vi "SQLite Select All SensorConfigValue_Old.vi"(6 "ALL/Single":T1(ring), 7 "Main":string="0", 8 "error in (no error)":errorcluster, 11 "SensorName":string) -> (0 "error out":errorcluster, 1 "SensorNameList":string[](array[string]), 2 "RowsNumber":string[](array[string]), 3 "Results":string[][](table), 5 "ColumnNames":string[](array[string]))   [LabVIEW 2015, in "SQLite.lvclass"]
doc: "读取Sensor的配置数据。\n2020-03-06 09:56:51\n蒋松\njiangsong@outlook.com"
uses:
  SQLite.lvclass
  SQLiteFileName.ctl
  TabelFullName.ctl
  <vilib>/Utility/error.llb/Trim Whitespace.vi
  <userlib>/sushu/sushu.lvlib
  <userlib>/LabSQL/LabSQL.lvlib
panel:
  out "resulting string":string
  out "OK？":bool
  out "Select SQL CMD":string
  out "String":string
  in  "error in (no error) 2":errorcluster
  # "8"
  # "8"
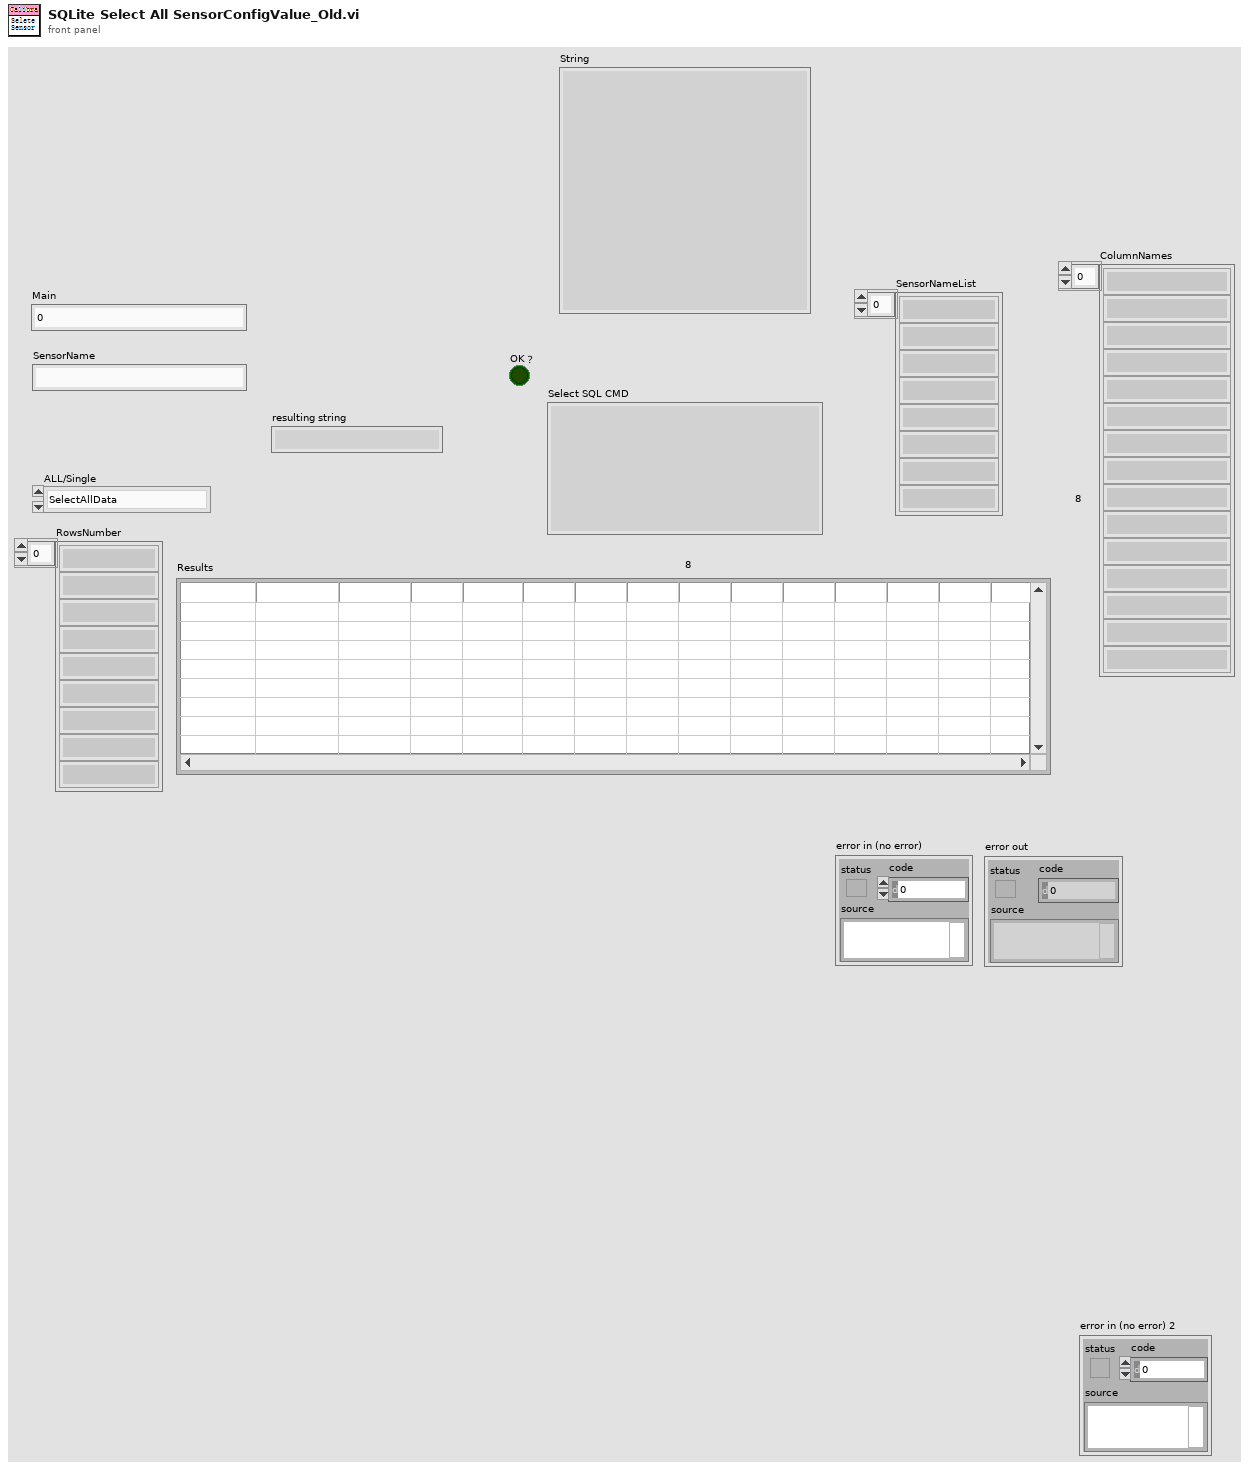
[diagram p1: front panel]
types:
  T1 = enum16{"SelectAllData", "SelectDataBySensorName"}
  T2 = typedef "SQLite.lvclass/TabelFullName.ctl" = string
  T3 = typedef "SQLite.lvclass/SQLiteFileName.ctl" = string
  T4 = enum16{"Other", "SQL2008", "SQLite", "Access", "MySQL"}
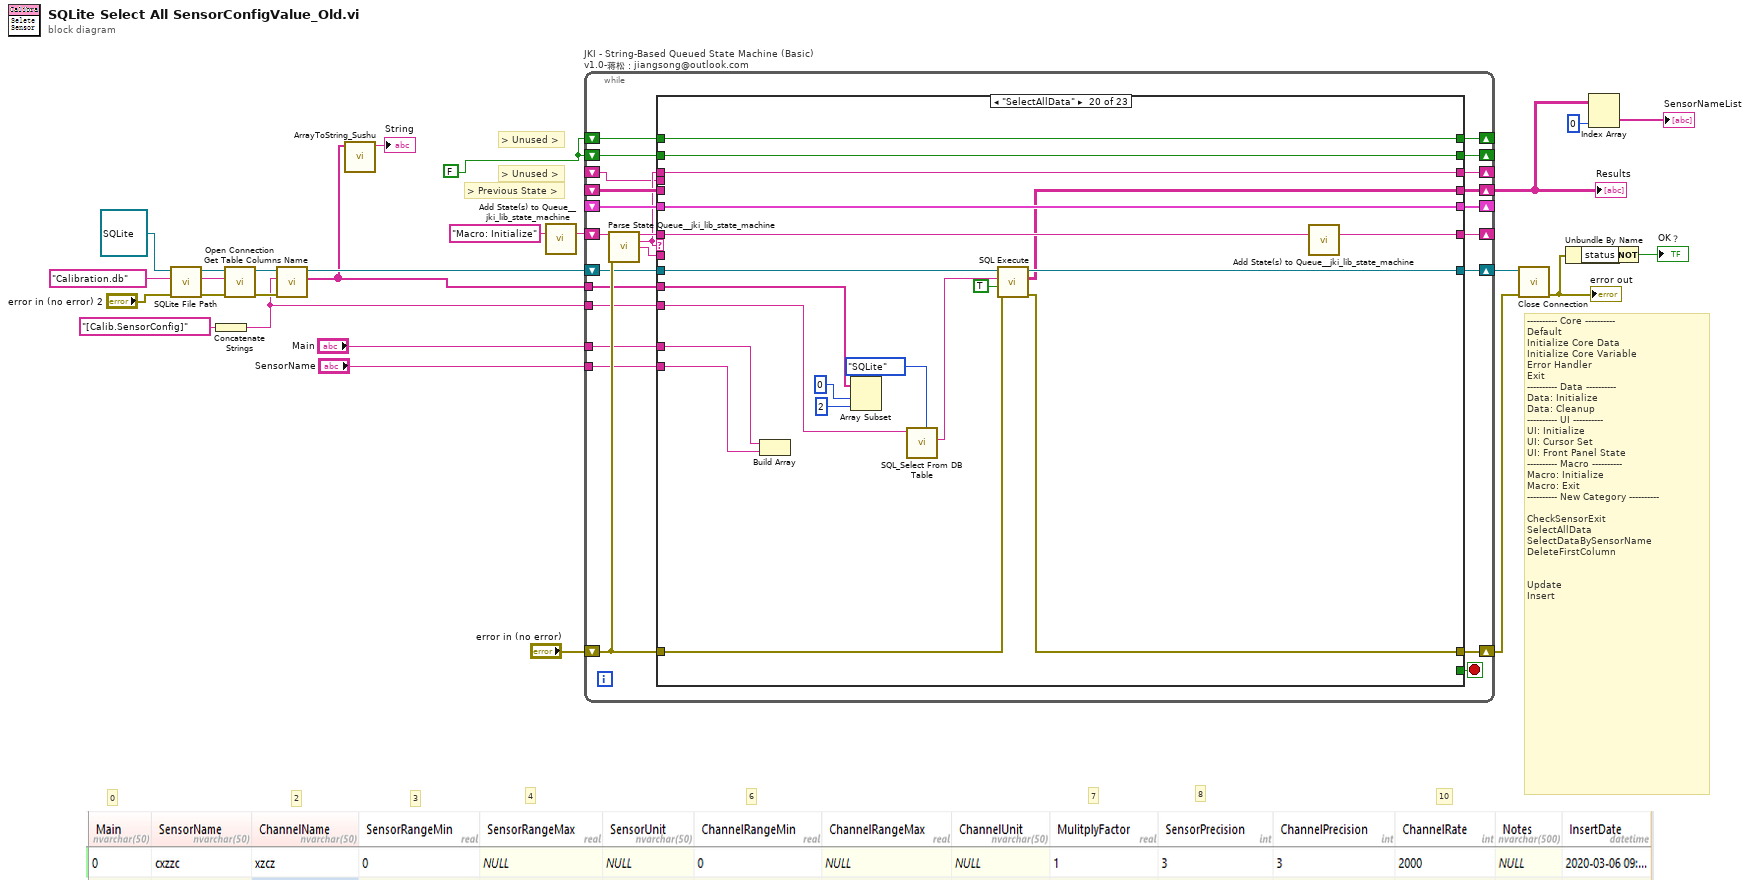
[diagram p0: block diagram]
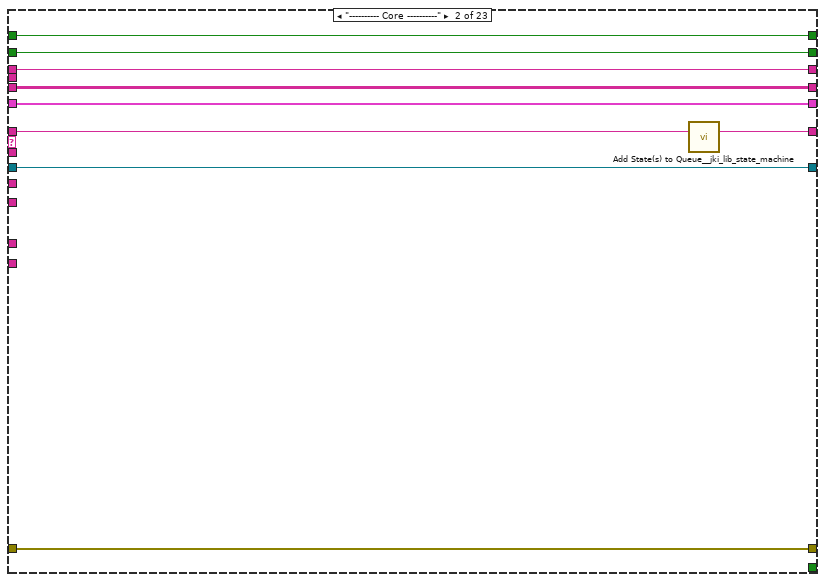
[diagram p3: hidden frame]
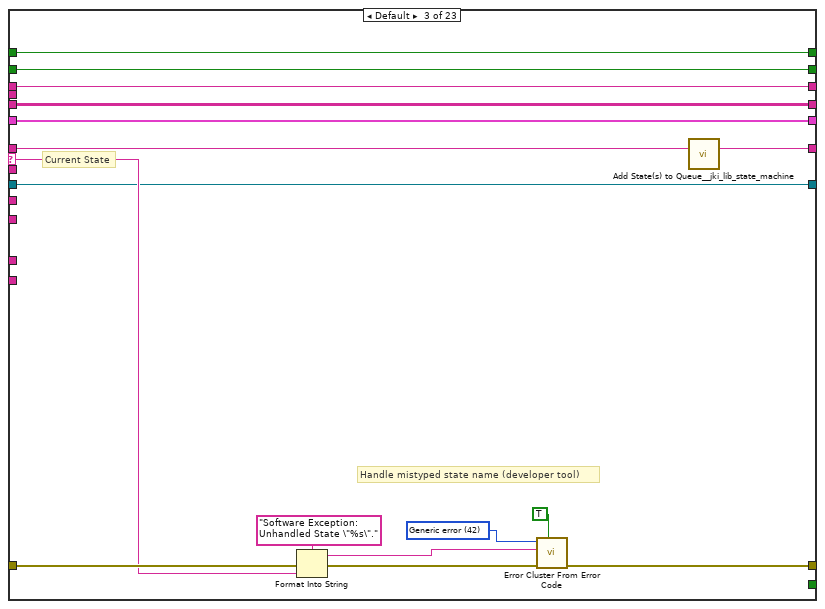
[diagram p4: hidden frame]
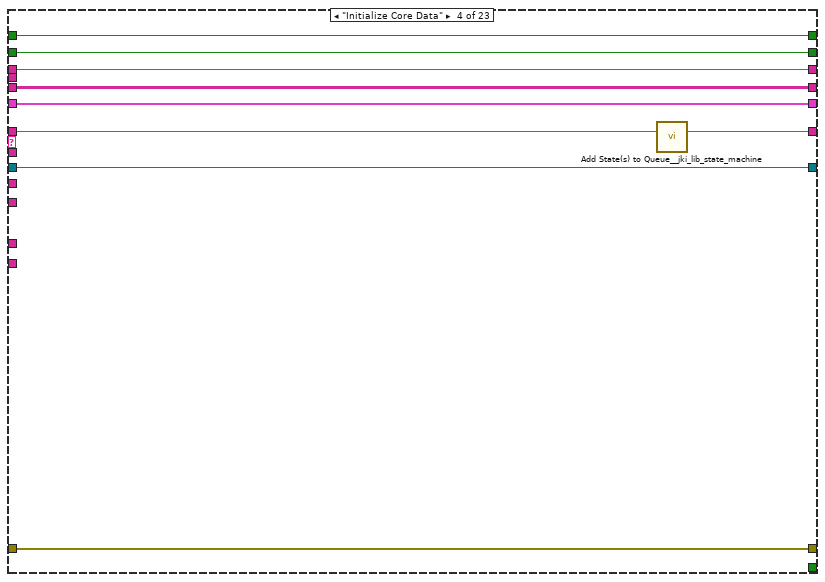
[diagram p5: hidden frame]
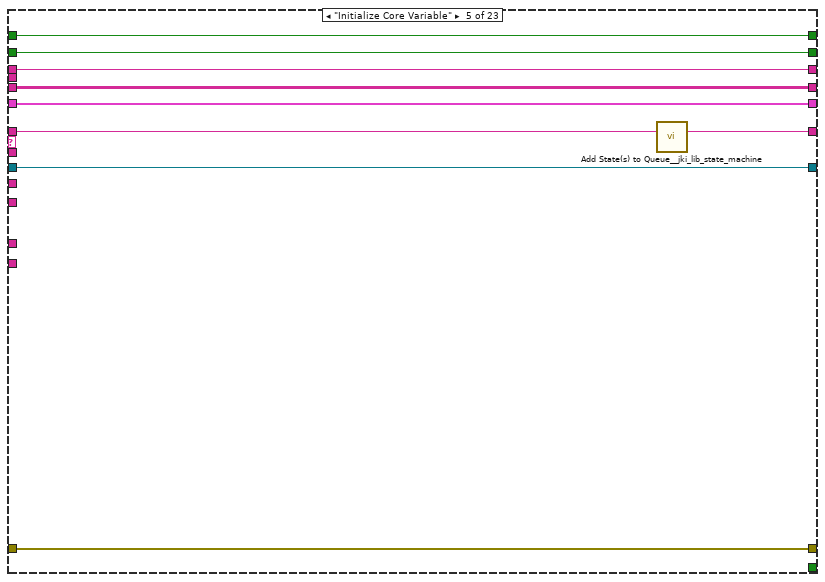
[diagram p6: hidden frame]
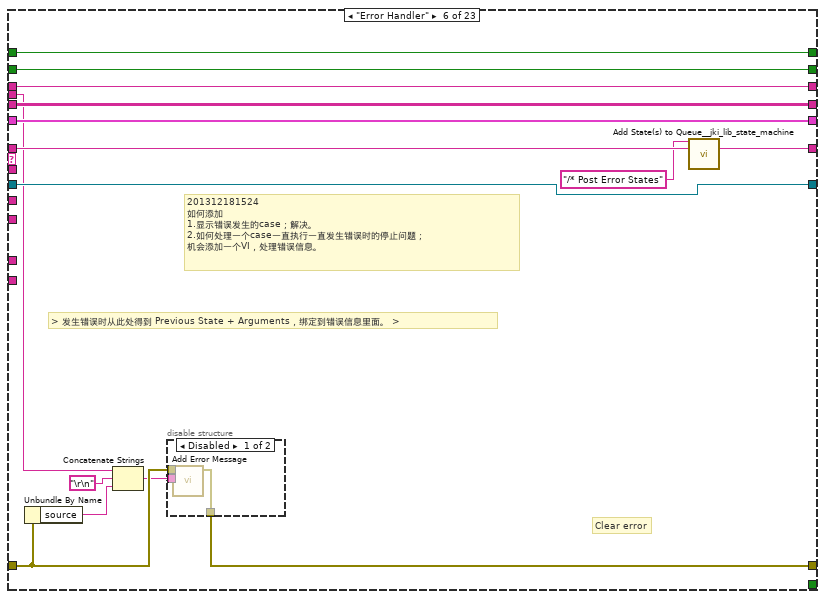
[diagram p7: hidden frame]
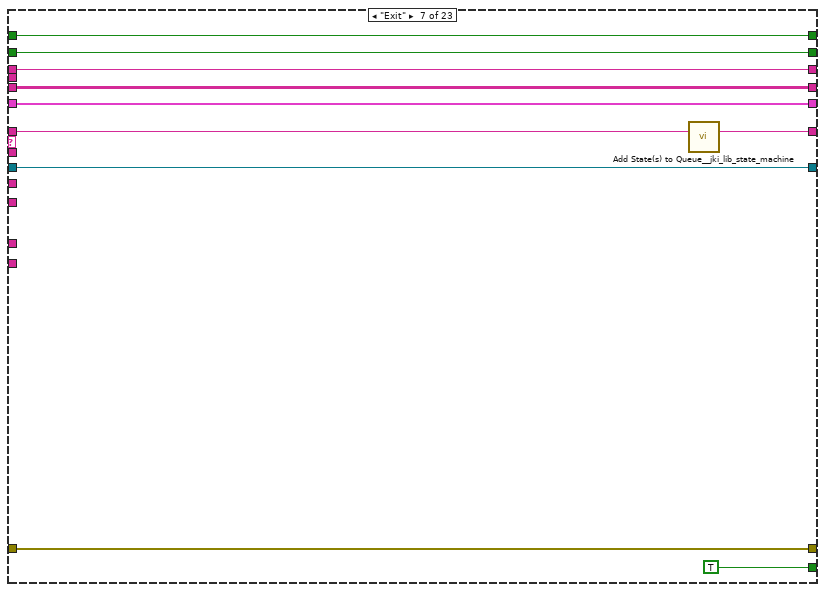
[diagram p9: hidden frame]
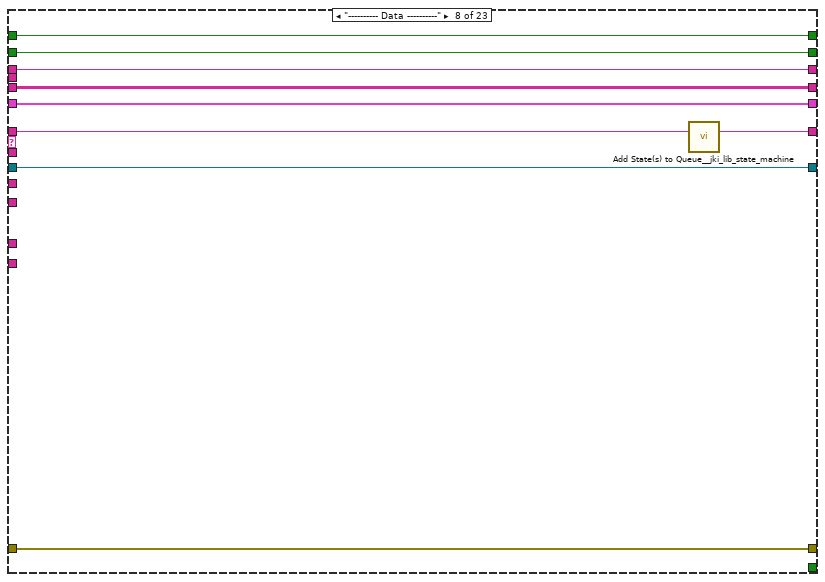
[diagram p10: hidden frame]
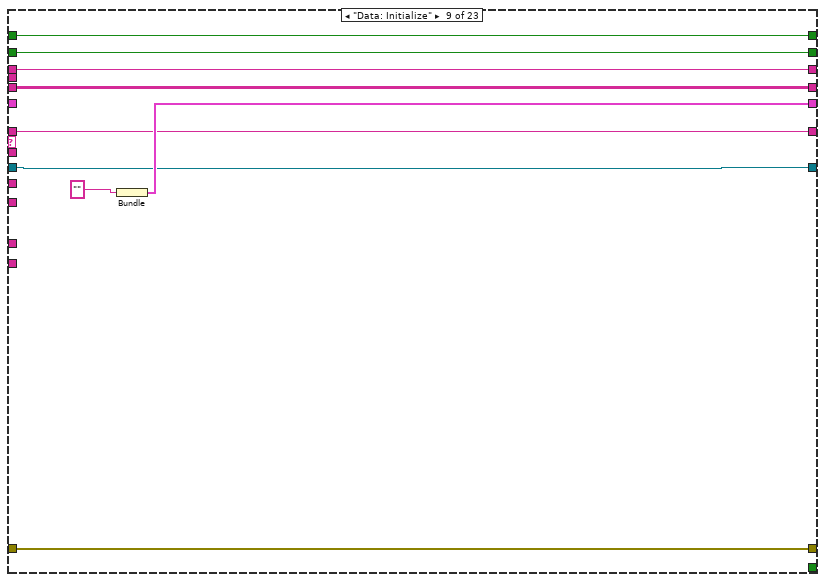
[diagram p11: hidden frame]
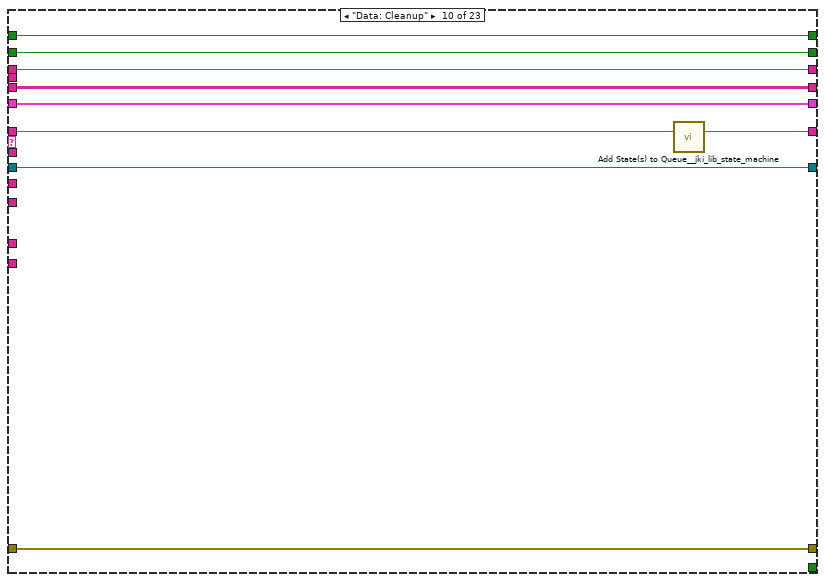
[diagram p12: hidden frame]
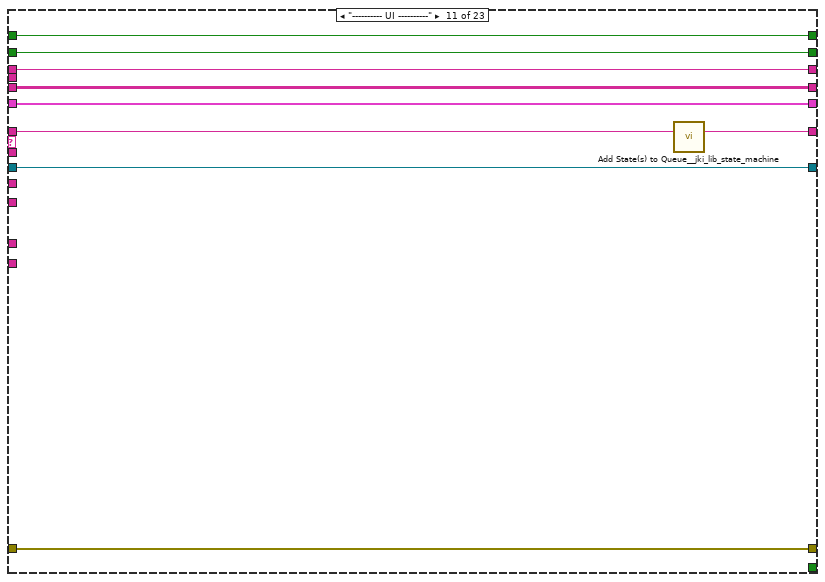
[diagram p13: hidden frame]
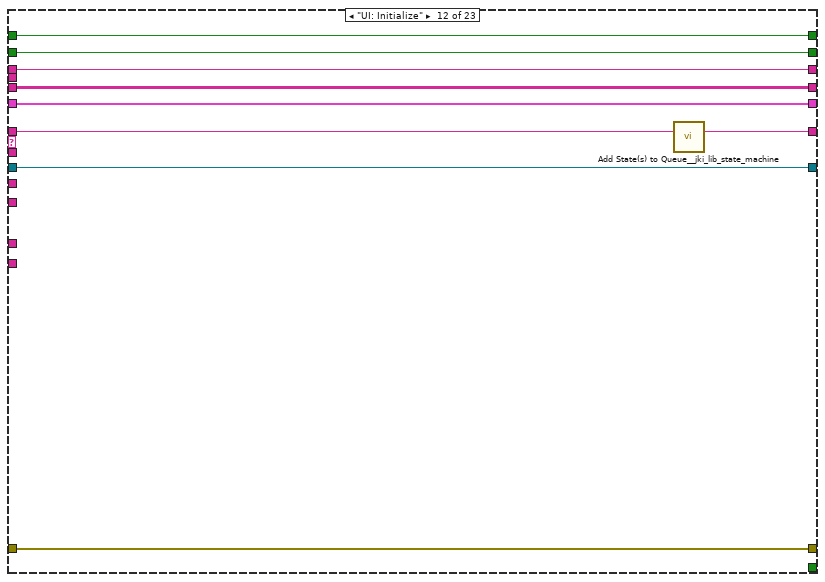
[diagram p14: hidden frame]
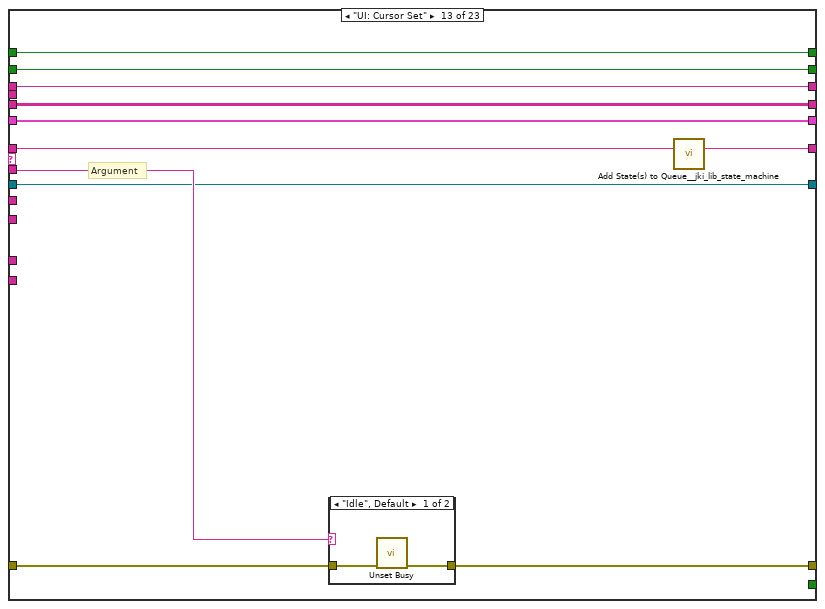
[diagram p15: hidden frame]
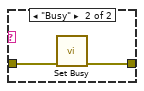
[diagram p16: hidden frame]
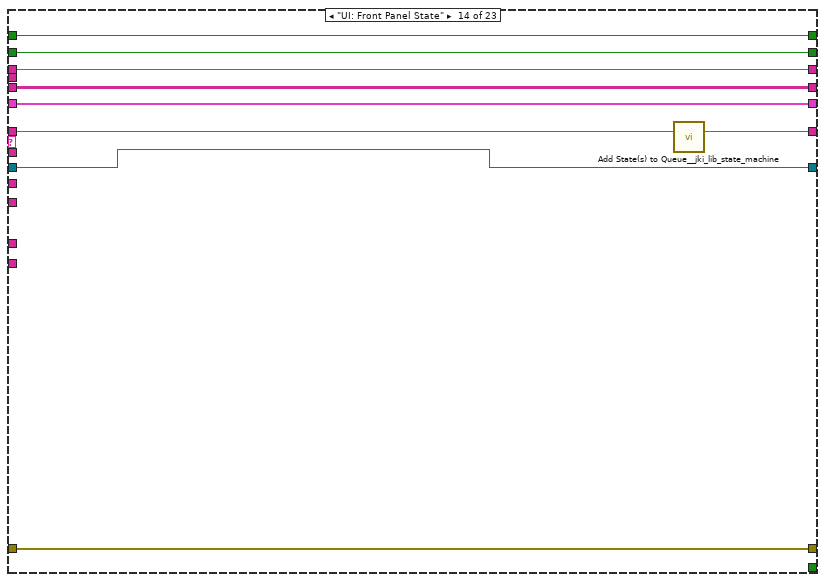
[diagram p17: hidden frame]
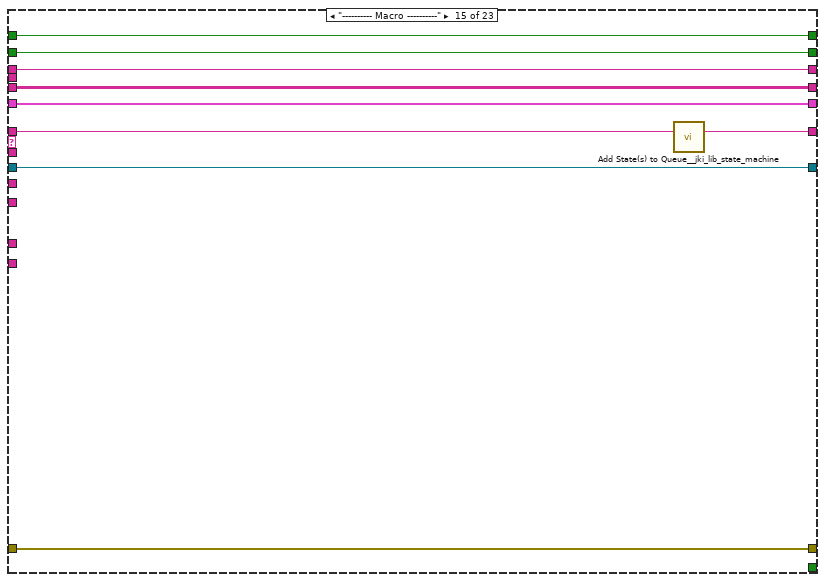
[diagram p18: hidden frame]
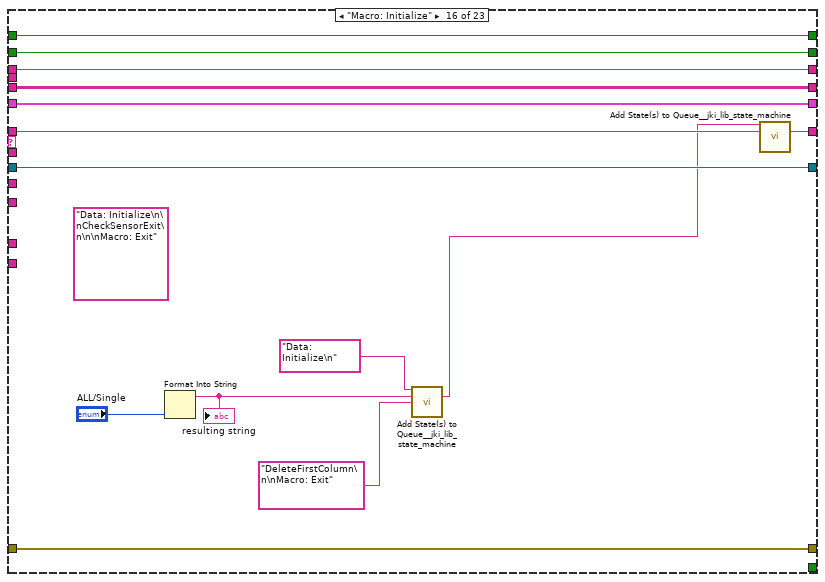
[diagram p19: hidden frame]
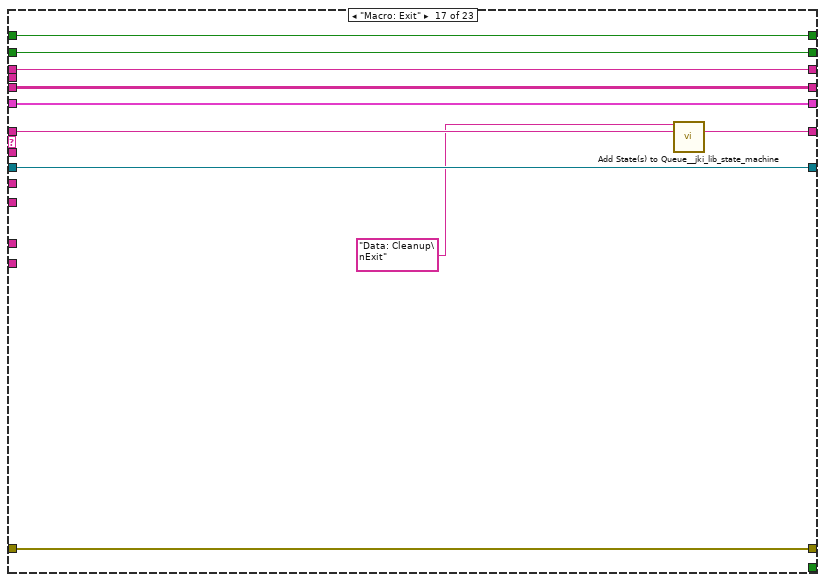
[diagram p20: hidden frame]
diagram:
  w4 = FALSE
  # "10"
  # "8"
  # "7"
  # "6"
  # "3"
  # "0"
  # "> Previous State >"
  # "> Unused >"
  # "> Unused >"
  # "---------- Core ----------\nDefault\nInitialize Core Data\nInitialize Core Variable\nError Handler\nExit\n---------- Data ----------\nData: Initialize\nData: Cleanup\n---------- UI ----------\nUI: Initialize\nUI: Cursor Set\nUI: Front Panel State\n---------- Macro ----------\nMacro: Initialize\nMacro: Exit\n---------- New Category ----------\n\nCheckSensorExit\nSelectAllData\nSelectDataBySensorName\nDeleteFirstColumn\n\n\nUpdate\nInsert"
  # "2"
  # "4"
  n1 = call "SQLite File Path.vi"("error in (no error)"="error in (no error) 2", "SQLiteFileName"=T3 "Calibration.db", "SQLite in"=refnum<class "SQLite.lvclass"> refnum ("SQLite.lvclass")) -> ("error out"=w22:errorcluster, "string"=w18:string, "SQLite out"=w20:refnum<class "SQLite.lvclass">)  [unwired: 6 in]
  n2 = Concatenate Strings(T2 "[Calib.SensorConfig]" ("TabelFullName")) -> (w13:string)
  n3 = call-dynamic "Open Connection.vi"("error in (no error)"=w22, "ConnectionString"=w18, "HostDB in"=w20) -> ("error out"=w17:errorcluster, "HostDB out"=w16:refnum<class "SQLite.lvclass">)  [unwired: 7 in]
  n4 = call-dynamic "Get Table Columns Name.vi"("error in (no error)"=w17, "TableName"=w13, "HostDB in"=w16) -> ("ColunmsList"=w9:string[], "HostDB out"=w14:refnum<class "SQLite.lvclass">)  [unwired: 4 in, 3 out]
  n5 = call <userlib>:"ArrayToString_Sushu.vi"("Array"=w9) -> ("String"=→"String":string)  [unwired: 10 in]
  n6 = call <vilib>:"Add State(s) to Queue__jki_lib_state_machine.vi"("State(s) in (\"\")"="Macro: Initialize") -> ("States Out"=w27:string)  [unwired: 14 in]
  n7 = while "JKI - String-Based Queued State Machine (Basic) v1.0-蒋松：jiangsong@outlook.com" {
    shift-right: [w49] -> w10
    shift-left: "error in (no error)" -> [w47]
    shift-right: [w30] -> _
    shift-left: w27 -> [w38]
    shift-right: [w43] -> _
    shift-left: w4 -> [w45]
    shift-right: [w44] -> _
    shift-left: w4 -> [w46]
    shift-right: [w39] -> _
    shift-left: _ -> [w42]
    shift-right: [w40] -> w3
    shift-left: _ -> [w31]
    shift-right: [w41] -> _
    shift-left: _ -> [w28]
    tunnel: w9 -> [w37]
    tunnel: w13 -> [w36]
    tunnel: "Main" -> [w35]
    tunnel: "SensorName" -> [w34]
    shift-right: [w32] -> w12
    shift-left: w14 -> [w33]
    stop <- w48 stop-if-true
    n8 = call <vilib>:"Parse State Queue__jki_lib_state_machine.vi"("State Queue"=w38, "Error In (no error)"=w47) -> ("Remaining States"=w51:string, "Current State"=w29:string, "Arguments"=w50:string)  [unwired: 11 in]
    n9 = case shown="\"SelectAllData\"" w29 {
      selector: w29 -> [_ _ w70 _ _ _ _ _ _ _ _ _ _ _ _ _ _ _ _ _ _ _ _]
      tunnel: w51 -> [w52 w68 w84 w93 w102 w117 w130 w139 w140 w157 w166 w175 w186 w199 w208 w214 w232 w241 w247 w269 w306 w332 w360]
      tunnel: w50 -> [_ _ _ _ _ _ _ _ _ _ _ _ w180 _ _ _ _ _ _ _ _ _ _]
      tunnel: [w59 w66 w71 w88 w100 w104 w123 w133 w145 w149 w160 w169 w178 w191 w202 w218 w227 w236 w245 w267 w307 w311 w335] -> w49
      tunnel: w47 -> [w59 w66 w72 w88 w100 w107 w123 w133 w145 w149 w160 w169 w179 w191 w202 w218 w227 w236 w246 w268 w307 w312 w336]
      tunnel: [w52 w67 w83 w92 w101 w116 w129 w138 w140 w156 w165 w174 w185 w198 w207 w215 w231 w240 w248 w270 w306 w332 w360] -> w30
      tunnel: [_ _ _ _ _ _ TRUE _ _ _ _ _ _ _ _ _ _ _ _ _ _ _ _] -> w48
      tunnel: w46 -> [w58 w65 w82 w91 w94 w115 w128 w137 w148 w155 w164 w173 w184 w197 w206 w222 w230 w239 w263 w283 w305 w331 w359]
      tunnel: w45 -> [w57 w64 w81 w90 w95 w114 w127 w136 w147 w154 w163 w172 w183 w196 w205 w221 w229 w238 w262 w282 w304 w330 w358]
      tunnel: [w58 w65 w82 w91 w94 w115 w128 w137 w148 w155 w164 w173 w184 w197 w206 w222 w230 w239 w263 w283 w305 w331 w359] -> w44
      tunnel: [w57 w64 w81 w90 w95 w114 w127 w136 w147 w154 w163 w172 w183 w196 w205 w221 w229 w238 w262 w282 w304 w330 w358] -> w43
      tunnel: w29 -> [w56 w63 w80 w89 w96 w113 w126 w135 w146 w153 w162 w171 w182 w195 w204 w220 w228 w237 w261 w281 w303 w329 w357]
      tunnel: w31 -> [w54 w61 w79 w87 w97 w110 w122 w132 w143 w151 w159 w168 w177 w193 w201 w217 w225 w234 _ _ w300 w328 w356]
      tunnel: w42 -> [w55 w62 w78 w85 w99 w105 w125 w134 _ w152 w161 w170 w181 w194 w203 w219 w226 w235 w260 w280 w302 w327 w355]
      tunnel: [w56 w63 w80 w89 w96 w113 w126 w135 w146 w153 w162 w171 w182 w195 w204 w220 w228 w237 w261 w281 w303 w329 w357] -> w41
      tunnel: [w54 w61 w79 w87 w97 w110 w122 w132 w143 w151 w159 w168 w177 w193 w201 w217 w225 w234 w244 w266 w287 w328 w356] -> w40
      tunnel: [w55 w62 w78 w85 w99 w105 w125 w134 w144 w152 w161 w170 w181 w194 w203 w219 w226 w235 w260 w280 w302 w327 w355] -> w39
      tunnel: w37 -> [_ _ _ _ _ _ _ _ _ _ _ _ _ _ _ _ _ _ w252 w274 w295 w319 w342]
      tunnel: w36 -> [_ _ _ _ _ _ _ _ _ _ _ _ _ _ _ _ _ _ w251 w273 _ w321 w348]
      tunnel: w35 -> [_ _ _ _ _ _ _ _ _ _ _ _ _ _ _ _ _ _ w250 w272 _ w326 w354]
      tunnel: w34 -> [_ _ _ _ _ _ _ _ _ _ _ _ _ _ _ _ _ _ w249 w271 _ w325 w353]
      tunnel: w33 -> [w53 w60 w69 w86 w98 w108 w121 w131 w142 w150 w158 w167 w176 w192 w200 w216 w224 w233 w254 w276 w301 w324 w352]
      tunnel: [w53 w60 w69 w86 w98 w108 w121 w131 w142 w150 w158 w167 w176 w192 w200 w216 w224 w233 w253 w275 w301 w323 w351] -> w32
      tunnel: w28 -> [_ _ _ _ _ w103 _ _ _ _ _ _ _ _ _ _ _ _ _ _ _ _ _]
      frame "Idle" {
      }
      frame "---------- Core ----------" {
        n10 = call <vilib>:"Add State(s) to Queue__jki_lib_state_machine.vi"("State(s) in (\"\")"=w68) -> ("States Out"=w67:string)  [unwired: 14 in]
      }
      frame Default {
        w74 = 42 items=["No error", "Argument error", "Memory is full", "Out of zone", "End of file", "File already open", "Generic file I/O error", "File not found", "File permission error", "Disk is full", "Duplicate path", "Too many files open", "System feature not enabled", "Resource file not found", "Cannot add resource", "Resource not found", "Image not found", "Image memory error", "Pen does not exist", "Config type invalid", "Config token not found", "Config parse error", "Config memory error", "Bad external code format", "Bad external code offset", "External code not present", "Null window", "Destroy window error", "Null menu", "Print aborted", "Bad print record", "Print driver error", "Windows error during printing", "Memory error during printing", "Print dialog error", "Generic print error", "Invalid device refnum", "Device not found", "Device parameter error", "Device unit error", "Cannot open device", "Device call aborted", "Generic error", "Cancelled by user", "Object ID too low", "Object ID too high", "Object not in heap", "Unknown heap", "Unknown object (invalid DefProc)", "Unknown object (DefProc not in table)", "Message out of range", "Invalid (null) method", "Unknown message", "Manager call not supported", "Bad address", "Network operation in progress", "Network operation timed out", "Connection is busy", "Network attribute not supported", "Network error", "Address in use", "System out of memory", "Connection aborted", "Connection refused", "Not connected", "Already connected", "Connection closed", "Initialization error (interapplication manager)", "Bad occurrence", "Wait on unbound occurrence handler", "Occurrence queue overflow", "Datalog type conflict", "Unused", "Unrecognized type (interapplication manager)", "Memory corrupt", "Failed to make temporary DLL", "Old CIN version", "Drag socket not found", "Failed to load drop-object", "Failed to register OLE object", "Failed to release OLE object", "Format specifier type mismatch", "Unknown format specifier", "Too few format specifiers", "Too many format specifiers", "Scan failed", "Newer CIN version", "Error converting to variant", "Runtime menu error", "Password tampered", "Variant attribute not found", "Incompatible variant data type", "Event data is not available", "Event Store is not present", "Occurrence is not found", "Event Queue is not created", "Event info is not available", "Refnum passed is NULL", "Error retrieving Class GUID", "Error retrieving CoClass GUID", "Error retrieving TypeLib GUID.", "Bad built application magic bytes.", "Specific driver is different from the specific driver associated with the Logical Name.", "There is no session opened to the class driver.", "Max Error", "MAX - Error with config objects", "MAX - Error loading configuration", "MAX - Group not supported"]
        # "Current State"
        # "Handle mistyped state name (developer tool)"
        n11 = Format Into String(format string="Software Exception: Unhandled State \"%s\"." ("message"), error in=w72, w70) -> (resulting string=w75:string, error out=w76:errorcluster)  [unwired: 1 in]
        n12 = call <vilib>:"Error Cluster From Error Code.vi"("show call chain? (False)"=TRUE, "error in (no error)"=w76, "error message (\"\")"=w75, "error code (0)"=w74) -> ("error out"=w71:errorcluster)  [unwired: 5 in]
        n13 = call <vilib>:"Add State(s) to Queue__jki_lib_state_machine.vi"("State(s) in (\"\")"=w84) -> ("States Out"=w83:string)  [unwired: 14 in]
      }
      frame "Initialize Core Data" {
        n14 = call <vilib>:"Add State(s) to Queue__jki_lib_state_machine.vi"("State(s) in (\"\")"=w93) -> ("States Out"=w92:string)  [unwired: 14 in]
      }
      frame "Initialize Core Variable" {
        n15 = call <vilib>:"Add State(s) to Queue__jki_lib_state_machine.vi"("State(s) in (\"\")"=w102) -> ("States Out"=w101:string)  [unwired: 14 in]
      }
      frame "Error Handler" {
        # "> 发生错误时从此处得到 Previous State + Arguments，绑定到错误信息里面。 >"
        # "201312181524\n如何添加\n1.显示错误发生的case；解决。\n2.如何处理一个case一直执行一直发生错误时的停止问题；\n机会添加一个VI，处理错误信息。"
        # "Clear error"
        n16 = Unbundle By Name(w107) -> ("source"=w109:string)
        n17 = Concatenate Strings(w103, "\r\n", w109) -> (w106:string)
        n18 = disable-structure shown="Disabled" {
          disable-tunnel: w107 -> [w120 _]
          disable-tunnel: w106 -> [w119 _]
          disable-tunnel: [w118 _] -> w104
          frame Disabled {
            n19 = call <userlib>:"Add Error Message.vi"("ErrorMessages"=w119, "error in (no error)"=w120) -> ("error out"=w118:errorcluster)  [unwired: 9 in]
          }
          frame Enabled {
          }
        }
        n20 = call <vilib>:"Add State(s) to Queue__jki_lib_state_machine.vi"("State(s) in Front (\"\")"="/* Post Error States", "State(s) in (\"\")"=w117) -> ("States Out"=w116:string)  [unwired: 13 in]
      }
      frame "Exit" {
        n21 = call <vilib>:"Add State(s) to Queue__jki_lib_state_machine.vi"("State(s) in (\"\")"=w130) -> ("States Out"=w129:string)  [unwired: 14 in]
      }
      frame "---------- Data ----------" {
        n22 = call <vilib>:"Add State(s) to Queue__jki_lib_state_machine.vi"("State(s) in (\"\")"=w139) -> ("States Out"=w138:string)  [unwired: 14 in]
      }
      frame "Data: Initialize" {
        n23 = Bundle("") -> (w144:cluster{string})  [unwired: 1 in]
      }
      frame "Data: Cleanup" {
        n24 = call <vilib>:"Add State(s) to Queue__jki_lib_state_machine.vi"("State(s) in (\"\")"=w157) -> ("States Out"=w156:string)  [unwired: 14 in]
      }
      frame "---------- UI ----------" {
        n25 = call <vilib>:"Add State(s) to Queue__jki_lib_state_machine.vi"("State(s) in (\"\")"=w166) -> ("States Out"=w165:string)  [unwired: 14 in]
      }
      frame "UI: Initialize" {
        n26 = call <vilib>:"Add State(s) to Queue__jki_lib_state_machine.vi"("State(s) in (\"\")"=w175) -> ("States Out"=w174:string)  [unwired: 14 in]
      }
      frame "UI: Cursor Set" {
        # "Argument"
        n27 = case shown="\"Idle\", Default" w180 {
          tunnel: w179 -> [w188 w190]
          tunnel: [w187 w189] -> w178
          frame "Idle", Default {
            n28 = call <vilib>:"Unset Busy.vi"("error in (no error)"=w188) -> ("error out"=w187:errorcluster)  [unwired: 10 in]
          }
          frame "Busy" {
            n29 = call <vilib>:"Set Busy.vi"("error in (no error)"=w190) -> ("error out"=w189:errorcluster)  [unwired: 9 in, 1 out]
          }
        }
        n30 = call <vilib>:"Add State(s) to Queue__jki_lib_state_machine.vi"("State(s) in (\"\")"=w186) -> ("States Out"=w185:string)  [unwired: 14 in]
      }
      frame "UI: Front Panel State" {
        n31 = call <vilib>:"Add State(s) to Queue__jki_lib_state_machine.vi"("State(s) in (\"\")"=w199) -> ("States Out"=w198:string)  [unwired: 14 in]
      }
      frame "---------- Macro ----------" {
        n32 = call <vilib>:"Add State(s) to Queue__jki_lib_state_machine.vi"("State(s) in (\"\")"=w208) -> ("States Out"=w207:string)  [unwired: 14 in]
      }
      frame "Macro: Initialize" {
        (unwired) "Data: Initialize\n\nCheckSensorExit\n\n\nMacro: Exit"
        n33 = Format Into String("ALL/Single") -> (resulting string=w211:string)  [unwired: 3 in, 1 out]
        "resulting string" <- w211
        n34 = call <vilib>:"Add State(s) to Queue__jki_lib_state_machine.vi"("State(s) in Front (\"\")"="Data: Initialize\n", "State(s) in (\"\")"=w211, "State(s) at Back (\"\")"="DeleteFirstColumn\n\nMacro: Exit") -> ("States Out"=w209:string)  [unwired: 12 in]
        n35 = call <vilib>:"Add State(s) to Queue__jki_lib_state_machine.vi"("State(s) in Front (\"\")"=w209, "State(s) in (\"\")"=w214) -> ("States Out"=w215:string)  [unwired: 13 in]
      }
      frame "Macro: Exit" {
        n36 = call <vilib>:"Add State(s) to Queue__jki_lib_state_machine.vi"("State(s) in Front (\"\")"="Data: Cleanup\nExit", "State(s) in (\"\")"=w232) -> ("States Out"=w231:string)  [unwired: 13 in]
      }
      frame "---------- New Category ----------" {
        n37 = call <vilib>:"Add State(s) to Queue__jki_lib_state_machine.vi"("State(s) in (\"\")"=w241) -> ("States Out"=w240:string)  [unwired: 14 in]
      }
      frame "SelectDataBySensorName" {
        n38 = Build Array(w250, w249) -> (w258:string[])
        n39 = Array Subset(array=w252, index=0, length=2) -> (w256:string[])
        n40 = call <userlib>:"SQL_Select From DB Table.vi"("DB Type"=T4."SQLite", "ColumnsValue"=w258, "ColumnsNameList"=w256, "TableName"=w251) -> ("Select SQL CMD"=w259:string)  [unwired: 7 in]
        "Select SQL CMD" <- w259
        n41 = call-dynamic "SQL Execute.vi"("error in (no error)"=w246, "Return Data (T)"=TRUE, "Command Text"=w259, "HostDB in"=w254) -> ("error out"=w245:errorcluster, "Table Control"=w244:string[][], "HostDB out"=w253:refnum<class "SQLite.lvclass">)  [unwired: 3 in, 2 out]
        n42 = call <vilib>:"Add State(s) to Queue__jki_lib_state_machine.vi"("State(s) in (\"\")"=w247) -> ("States Out"=w248:string)  [unwired: 14 in]
      }
      frame "SelectAllData" {
        n43 = Build Array(w272, w271) -> ()  [unwired: 1 out]
        n44 = Array Subset(array=w274, index=0, length=2) -> ()  [unwired: 1 out]
        n45 = call <userlib>:"SQL_Select From DB Table.vi"("DB Type"=T4."SQLite", "TableName"=w273) -> ("Select SQL CMD"=w279:string)  [unwired: 9 in]
        n46 = call-dynamic "SQL Execute.vi"("error in (no error)"=w268, "Return Data (T)"=TRUE, "Command Text"=w279, "HostDB in"=w276) -> ("error out"=w267:errorcluster, "Table Control"=w266:string[][], "HostDB out"=w275:refnum<class "SQLite.lvclass">)  [unwired: 3 in, 2 out]
        n47 = call <vilib>:"Add State(s) to Queue__jki_lib_state_machine.vi"("State(s) in (\"\")"=w269) -> ("States Out"=w270:string)  [unwired: 14 in]
      }
      frame "DeleteFirstColumn" {
        w290 = 0 ("disabled index (col)")
        w294 = 1 ("length")
        # "deletet the first column"
        # "delete the end column, datetime"
        n48 = Delete From Array(array=w300, length=w294, index (col)=w290) -> (array with subset deleted=w299:string[][])  [unwired: 1 in, 1 out]
        n49 = Array Size(array=w299) -> (size(s)=w298:i32[])
        n50 = Delete From Array(array=w295, length=w294, index=w290) -> (array with subset deleted=w293:string[])  [unwired: 1 out]
        n51 = Index Array(array=w298) -> (element #2=w297:i32)  [unwired: 2 in, 1 out]
        n52 = Array Size(array=w293) -> (size(s)=w292:i32)
        n53 = Decrement(x=w297) -> (x-1=w296:i32)
        n54 = Delete From Array(array=w299, length=w294, index (col)=w296) -> (array with subset deleted=w287:string[][])  [unwired: 1 in, 1 out]
        n55 = Decrement(x=w292) -> (x-1=w291:i32)
        n56 = Array Size(array=w287) -> (size(s)=w288:i32[])
        n57 = Delete From Array(array=w293, length=1, index=w291) -> (array with subset deleted=→"ColumnNames":string[])  [unwired: 1 out]
        n58 = Index Array(array=w288) -> (element=w285:i32)  [unwired: 1 in]
        n59 = for {
          N: w285 -> [_]
          tunnel: [w308] -> w286 mode=indexing
          i -> [w310]
          n60 = Increment(x=w310) -> (x+1=w309:i32)
          n61 = Number To Decimal String(number=w309) -> (decimal integer string=w308:string)  [unwired: 1 in]
        }
        "RowsNumber" <- w286
      }
      frame "Insert" {
        n62 = disable-structure shown="Disabled" {
          disable-tunnel: [w333 _] -> w316
          frame Disabled {
            n63 = call <userlib>:"StringToArray_Sushu.vi"() -> ("Array"=w333:string[])  [unwired: 10 in, 1 out]
          }
          frame Enabled {
          }
        }
        n64 = Build Array (concatenate)(w326, w325, w316) -> (w315:string[])
        n65 = Array Size(array=w315) -> (size(s)=w314:i32)
        n66 = Array Subset(array=w319, index=0, length=w314) -> (w320:string[])
        n67 = call <userlib>:"SQL_Insert DB Table.vi"("DB Type"=enum16{"Other", "SQL2008", "SQLite"}."SQLite", "ColumnsValue"=w315, "ColumnsName"=w320, "Table Name"=w321) -> ("Insert DB String"=w313:string)  [unwired: 7 in]
        n68 = call-dynamic "SQL Execute.vi"("error in (no error)"=w312, "Return Data (T)"=FALSE, "Command Text"=w313, "HostDB in"=w324) -> ("error out"=w311:errorcluster, "HostDB out"=w323:refnum<class "SQLite.lvclass">)  [unwired: 3 in, 3 out]
      }
      frame "Update" {
        n69 = call <userlib>:"StringToArray_Sushu.vi"() -> ("Array"=w337:string[])  [unwired: 10 in, 1 out]
        n70 = Build Array(w354, w353) -> (w344:string[])
        n71 = Array Subset(array=w342, index=0, length=2) -> (w340:string[])
        n72 = call <userlib>:"Build string_ColumnsName=ColumnsValue_Where and.vi"("DB Type"=T4."SQLite", "ColumnsValue"=w344, "Check ASCII?"=FALSE, "ColumnsNameList"=w340) -> ("ColumnName='ColumnValue'"=w338:string)  [unwired: 7 in]
        n73 = Array Size(array=w337) -> (size(s)=w345:i32)
        n74 = Array Subset(array=w342, index=2, length=w345) -> (w347:string[])
        n75 = call <userlib>:"SQL_Update DB Table.vi"("where name='value'"=w338, "ColumnsValue"=w337, "ColumnsNameList"=w347, "TableName"=w348) -> ("Update CMD"=w349:string)  [unwired: 7 in]
        n76 = call-dynamic "SQL Execute.vi"("error in (no error)"=w336, "Return Data (T)"=FALSE, "Command Text"=w349, "HostDB in"=w352) -> ("error out"=w335:errorcluster, "HostDB out"=w351:refnum<class "SQLite.lvclass">)  [unwired: 3 in, 3 out]
      }
    }
  }
  "Results" <- w3
  n77 = call-dynamic "Close Connection.vi"("error in (no error)"=w10, "HostDB in"=w12) -> ("error out"=w7:errorcluster)  [unwired: 8 in, 1 out]
  "error out" <- w7
  n78 = Unbundle By Name(w7) -> ("status"=w6:bool)
  n79 = Index Array(array=w3, index (col)=0 ("disabled index (col)")) -> (element=→"SensorNameList":string[])  [unwired: 1 in]
  n80 = Not(x=w6) -> (.not. x?=→"OK？":bool)
